vi "SSL_CTX_check_private_key.vi"(8 "error in (no error)":errorcluster, 11 "SSL-Context in":refnum<class "SSL-Context.lvclass">) -> (0 "error out":errorcluster, 3 "SSL-Context out":refnum<class "SSL-Context.lvclass">)   [LabVIEW 2013, in "OpenSSL Socket.lvlib" / "SSL-Context.lvclass"]
uses:
  SSL-Context.lvclass
  SSL-Lib/SSL-Lib.lvclass/SSL-Lib.ctl
  SSL-Context.lvclass/SSL-Context.ctl
  SSL-Lib/Read SSL Library Path.vi
  Read Handle.vi
  SSL-Lib/SSL-Lib.lvclass
panel:
  out "return type":i32
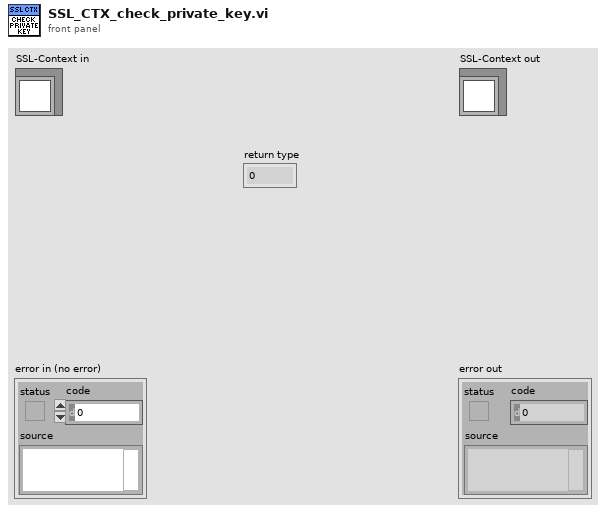
[diagram p1: front panel]
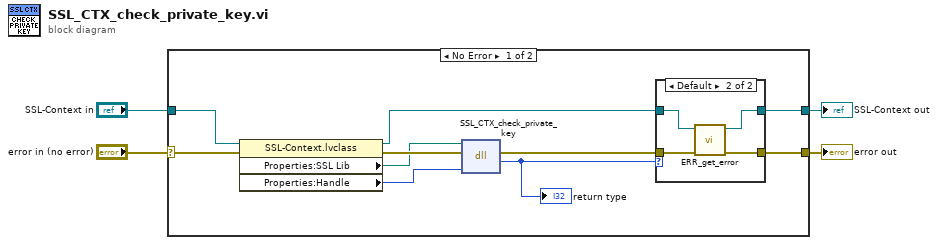
[diagram p0: block diagram]
diagram:
  n1 = case shown="No Error" "error in (no error)" {
    selector: "error in (no error)" -> [w14 w22]
    tunnel: [w6 w22] -> w3
    tunnel: [w7 w21] -> w1
    tunnel: "SSL-Context in" -> [w12 w21]
    frame No Error {
      n2 = property class="SSL-Context.lvclass"(reference=w12, error in=w14) -> (reference out=w8:refnum<class "SSL-Context.lvclass">, error out=w13:errorcluster, "Properties:SSL Lib"=w11:path, "Properties:Handle"=w10:u64)
      n3 = dll-call lib="C:/Program Files (x86)/National Instruments/Shared/nissl/NIssleay32.dll" fn="SSL_CTX_check_private_key"(path in=w11, error in=w13, "SSL_CTX"=w10) -> (error out=w9:errorcluster, "return type"=w5:i32)  [unwired: 2 in, 1 out]
      "return type" <- w5
      n4 = case shown="Default" w5 {
        tunnel: w9 -> [w16 w20]
        tunnel: w8 -> [w15 w19]
        tunnel: [w15 w18] -> w7
        tunnel: [w16 w17] -> w6
        frame 1 {
        }
        frame Default {
          n5 = call "ERR_get_error.vi"("error in (no error)"=w20, "SSL-Lib in"=w19) -> ("error out"=w17:errorcluster, "SSL-Lib out"=w18:refnum<class "SSL-Context.lvclass">)  [unwired: 8 in]
        }
      }
    }
    frame Error {
    }
  }
  "error out" <- w3
  "SSL-Context out" <- w1
